vi "barometer.vi"() -> ()   [LabVIEW 2014]
panel:
  out "PSI":dbl
  out "Pascals":i32
  out "InHg":i32
  out "Barometer":dbl(slide) scale=0.0..100.0
  in  "x*y":dbl=0.0168 step=0.001 format="%#_13g"
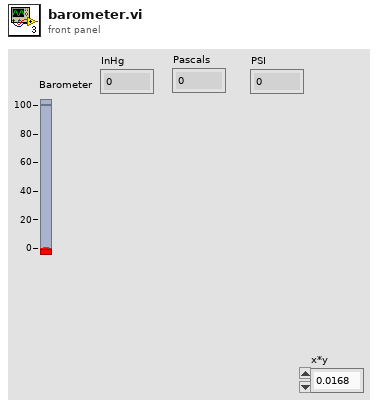
[diagram p1: front panel]
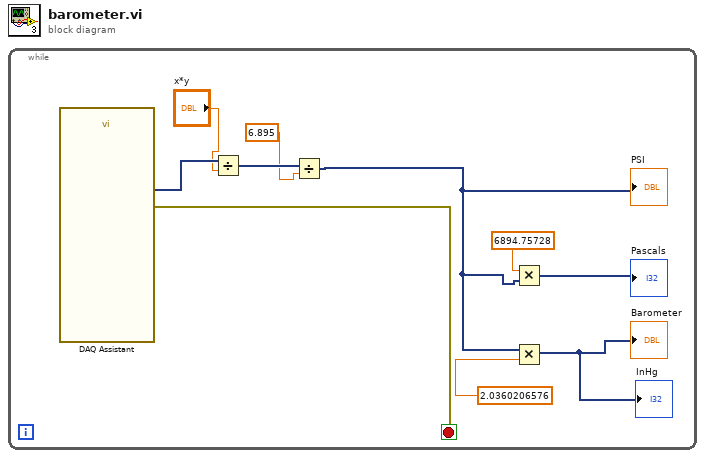
[diagram p0: block diagram]
diagram:
  n1 = while {
    stop <- w10 stop-if-true
    n2 = call "DAQ Assistant"() -> ("data"=w9:dynamicdata, "error out"=w10:errorcluster)  [unwired: 17 in, 1 out]
    n3 = Divide(x=w9, y="x*y") -> (x/y=w7:dynamicdata)
    n4 = Divide(x=w7, y=6.895 ("x")) -> (x/y=w1:dynamicdata)
    "PSI" <- w1
    n5 = Multiply(x=6894.75728, y=w1) -> (x*y=→"Pascals":dynamicdata)
    n6 = Multiply(x=w1, y=2.0360206576) -> (x*y=→"Barometer" →"InHg":dynamicdata)
  }
